vi "Configure Trigger Coupling.vi"(8 "error in (no error)":errorcluster, 9 "Trigger Coupling (0: DC)":u16(ring) items=["DC", "AC", "LFREJ", "HFREJ"], 10 "Trigger Source (1: Channel 1)":u16(ring)=1 items=["Channel 1"=1, "Channel 2"=2, "Channel 3"=3, "Channel 4"=4, "Ext"=5, "Ext5"=6, "AC Line"=7], 11 "VISA resource name":refnum<visa-resource-name>) -> (0 "error out":errorcluster, 3 "VISA resource name out":refnum<visa-resource-name>)   [LabVIEW 2021, in "Siglent SDS 1000 2000 Series.lvlib"]
doc: "Sets the coupling mode of the specified trigger source."
uses:
  <instrlib>/Siglent SDS 1000 2000 Series/Siglent SDS 1000 2000 Series.lvlib
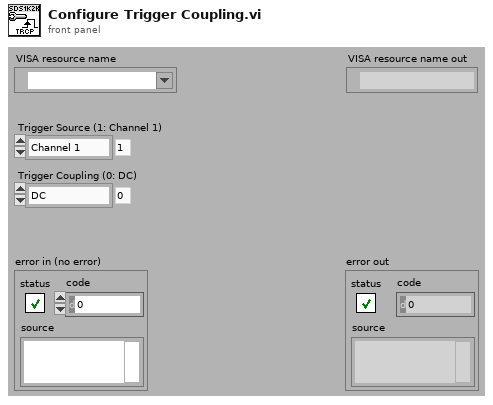
[diagram p1: front panel]
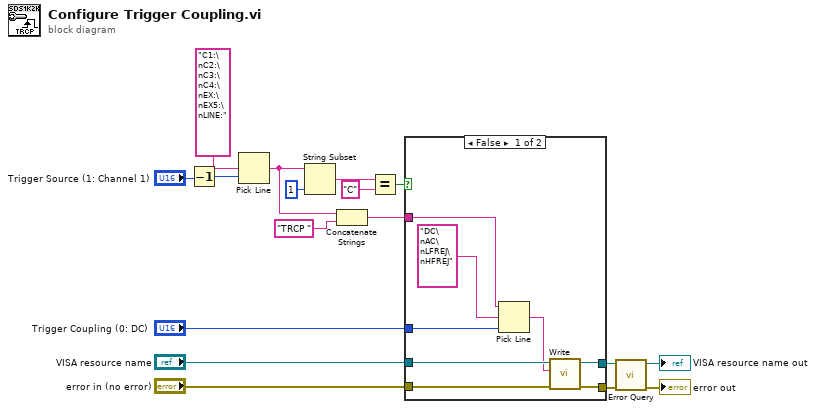
[diagram p0: block diagram]
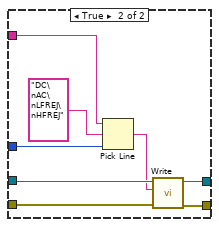
[diagram p2: hidden frame]
diagram:
  n1 = Decrement(x="Trigger Source (1: Channel 1)") -> (x-1=w1:u16)
  n2 = Pick Line(multi-line string="C1:\nC2:\nC3:\nC4:\nEX:\nEX5:\nLINE:", line index=w1) -> (output string=w5:string)  [unwired: 1 in]
  n3 = String Subset(string=w5, length (rest)=1 ("length (rest)")) -> (substring=w15:string)  [unwired: 1 in]
  n4 = Concatenate Strings(w5, "TRCP ") -> (w3:string)
  n5 = Equal?(x=w15, y="C") -> (x = y?=w13:bool)
  n6 = case shown="False" w13 {
    tunnel: [w23 w33] -> w9
    tunnel: [w22 w32] -> w6
    tunnel: w3 -> [w19 w29]
    tunnel: "VISA resource name" -> [w25 w31]
    tunnel: "error in (no error)" -> [w24 w30]
    tunnel: "Trigger Coupling (0: DC)" -> [w21 w26]
    frame False {
      n7 = Pick Line(string ("")=w19, multi-line string="DC\nAC\nLFREJ\nHFREJ", line index=w21) -> (output string=w20:string)
      n8 = call <instrlib>:"Write.vi"("error in (no error)"=w24, "Write Buffer"=w20, "VISA resource name"=w25) -> ("error out"=w22:errorcluster, "VISA resource name out"=w23:refnum<visa-resource-name>)  [unwired: 6 in, 1 out]
    }
    frame True {
      n9 = Pick Line(string ("")=w29, multi-line string="DC\nAC\nLFREJ\nHFREJ", line index=w26) -> (output string=w28:string)
      n10 = call <instrlib>:"Write.vi"("error in (no error)"=w30, "Write Buffer"=w28, "VISA resource name"=w31) -> ("error out"=w32:errorcluster, "VISA resource name out"=w33:refnum<visa-resource-name>)  [unwired: 6 in, 1 out]
    }
  }
  n11 = call <instrlib>:"Error Query.vi"("error in (no error)"=w6, "VISA resource name"=w9) -> ("error out"=→"error out":errorcluster, "VISA resource name out"=→"VISA resource name out":refnum<visa-resource-name>)  [unwired: 6 in, 2 out]
